vi "Valor de Modulacion Debugging Enviado.vi"(8 "error in (no error)":errorcluster, 9 "Nombre":string, 10 "Valor":dbl) -> (0 "error out":errorcluster)   [LabVIEW 2020, in "Pruebas.lvlib"]
doc: "Valor de Modulacion Debugging Enviado\n_____\nCreated using Delacor QMH Event Scripter 5.0.0.112."
uses:
  Pruebas.lvlib
  Valor de Modulacion Debugging Enviado Argument--cluster.ctl
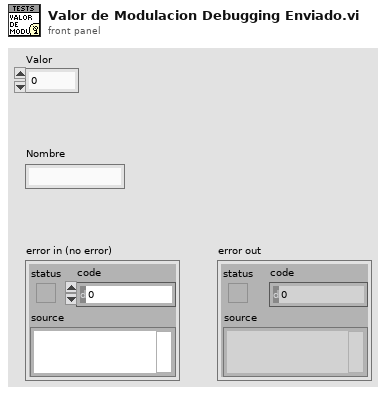
[diagram p1: front panel]
types:
  T1 = typedef "Pruebas.lvlib/Valor de Modulacion Debugging Enviado Argument--cluster.ctl" = cluster{"Valor":dbl, "Nombre":string}
  T2 = typedef "Pruebas.lvlib/Broadcast Events--cluster.ctl" = cluster{"Module Did Init":refnum<user-event>, "Status Updated":refnum<user-event>, "Error Reported":refnum<user-event>, "Module Did Stop":refnum<user-event>, "Update Module Execution Status":refnum<user-event>, "Controles de relés de prueba actualizados":refnum<user-event>, "Valor de Medicion de Prueba Enviado":refnum<user-event>, "Valor de Modulacion Debugging Enviado":refnum<user-event>}
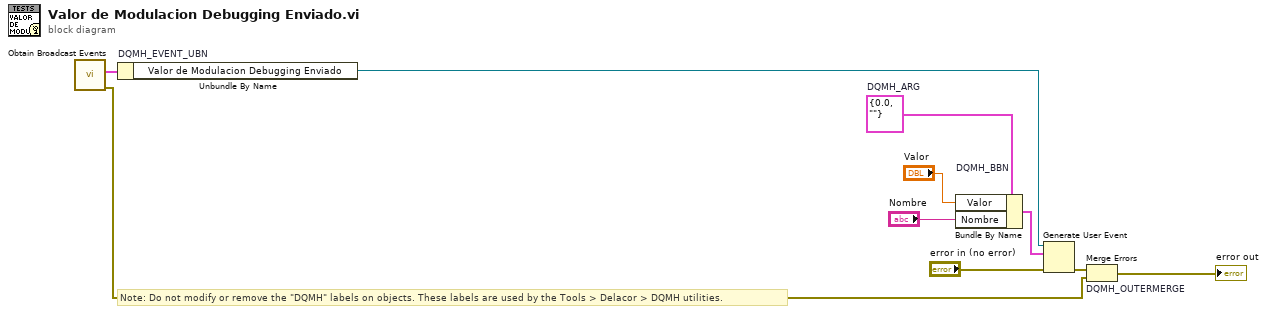
[diagram p0: block diagram]
diagram:
  w5 = T1 {"Valor"=0.0, "Nombre"=""}  # DQMH_ARG
  # "Note: Do not modify or remove the \"DQMH\" labels on objects. These labels are used by the Tools > Delacor > DQMH utilities."
  n1 = call "Obtain Broadcast Events.vi"() -> ("error out"=w2:errorcluster, "Pruebas Broadcast Events"=w1:T2)  [unwired: 10 in]
  n2 = Unbundle By Name "DQMH_EVENT_UBN"(w1) -> ("Valor de Modulacion Debugging Enviado"=w7:refnum<user-event>)
  n3 = Bundle By Name "DQMH_BBN"(cluster=w5, "Valor"="Valor", "Nombre"="Nombre") -> (w8:T1)
  n4 = Generate User Event(user event=w7, event data cluster=w8, error in="error in (no error)") -> (error out=w6:errorcluster)  [unwired: 1 in, 1 out]
  n5 = Merge Errors "DQMH_OUTERMERGE"(w6, w2) -> (→"error out":errorcluster)
